vi "TxtToExcel v3.vi"() -> ()   [LabVIEW 2016]
panel:
  out "output array":string[][](array[string])
  out "error out":errorcluster
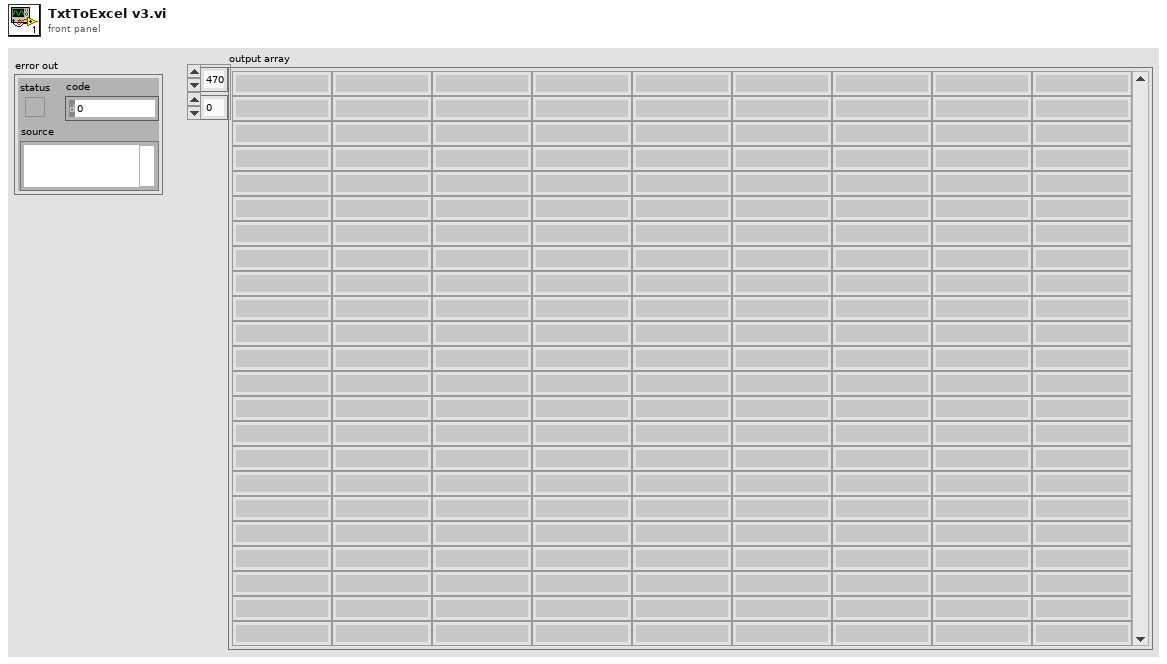
[diagram p1: front panel]
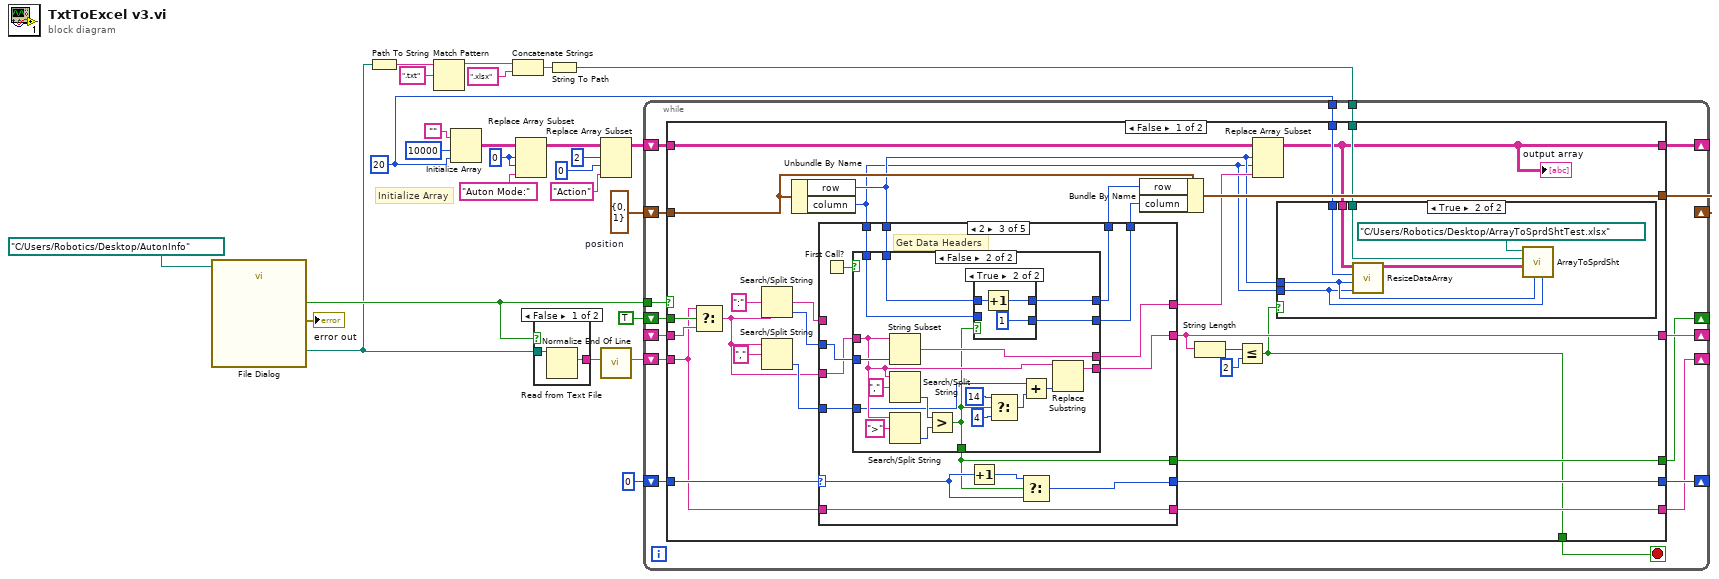
[diagram p0: block diagram]
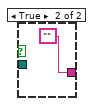
[diagram p2: hidden frame]
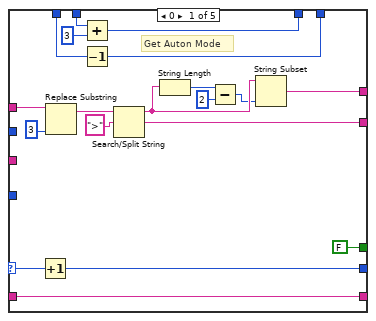
[diagram p4: hidden frame]
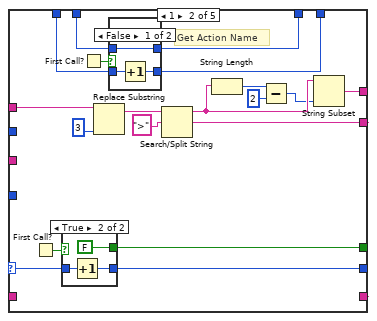
[diagram p5: hidden frame]
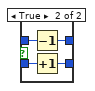
[diagram p6: hidden frame]
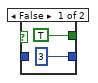
[diagram p7: hidden frame]
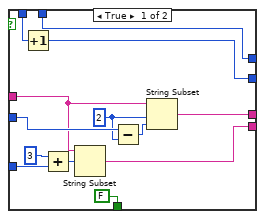
[diagram p8: hidden frame]
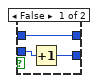
[diagram p9: hidden frame]
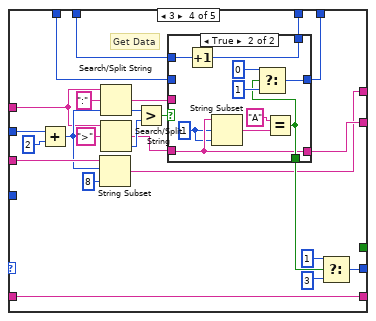
[diagram p10: hidden frame]
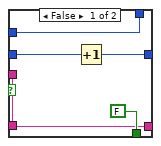
[diagram p11: hidden frame]
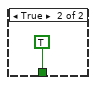
[diagram p13: hidden frame]
diagram:
  w15 = 0 ("index (row)")
  w17 = cluster{"row":i32, "column":i32} {"row"=0, "column"=1}  # position
  w1 = 20 ("Column Max")
  # "Initialize Array"
  n1 = call "File Dialog"("start path"=path "C:/Users/Robotics/Desktop/AutonInfo") -> ("selected path"=w8:path, "cancelled"=w24:bool, "error out"=→"error out":errorcluster)  [unwired: 11 in, 1 out]
  n2 = Path To String(path=w8) -> (string=w7:string)
  n3 = Match Pattern(string=w7, regular expression=".txt") -> (before substring=w3:string)  [unwired: 1 in, 3 out]
  n4 = Initialize Array("", 10000 ("Row Max"), w1) -> (w16:string[][])
  n5 = Concatenate Strings(w3, ".xlsx" ("string")) -> (w5:string)
  n6 = Replace Array Subset(array=w16, new element="Auton Mode:" ("new element/subarray"), index (row)=w15, index (col)=w15) -> (w13:string[][])
  n7 = case shown="False" w24 {
    tunnel: w8 -> [w28 _]
    tunnel: [w27 ""] -> w21
    frame False {
      n8 = Read from Text File(file (use dialog)=w28) -> (text=w27:string)  [unwired: 3 in, 3 out]
    }
    frame True {
    }
  }
  n9 = String To Path(string=w5) -> (path=w4:path)
  n10 = Replace Array Subset(array=w13, new element="Action" ("new element/subarray"), index (row)=2, index (col)=0 ("disabled index (col)")) -> (w9:string[][])
  n11 = call <vilib>:"Normalize End Of Line.vi"("string in"=w21) -> ("string out"=w20:string)  [unwired: 7 in]
  n12 = while {
    tunnel: w24 -> [w45]
    shift-right: [w42] -> _
    shift-left: _ -> [w44]
    shift-right: [w40] -> _
    shift-left: 0 -> [w41]
    shift-right: [w38] -> _
    shift-left: TRUE -> [w39]
    shift-right: [w37] -> _
    shift-left: w20 -> [w36]
    shift-right: [w32] -> _
    shift-left: w9 -> [w34]
    shift-right: [w33] -> _
    shift-left: w17 -> [w35]
    tunnel: w4 -> [w31]
    tunnel: w1 -> [w30]
    stop <- w43 stop-if-true
    n13 = case shown="False" w45 {
      tunnel: w44 -> [w66 _]
      tunnel: [w51 TRUE] -> w43
      tunnel: [w62 _] -> w42
      tunnel: w41 -> [w70 _]
      tunnel: [w69 _] -> w40
      tunnel: w39 -> [w64 _]
      tunnel: [w63 _] -> w38
      tunnel: [w59 _] -> w37
      tunnel: w36 -> [w58 _]
      tunnel: w35 -> [w56 _]
      tunnel: w34 -> [w55 _]
      tunnel: [w57 _] -> w33
      tunnel: [w46 _] -> w32
      tunnel: w31 -> [w50 _]
      tunnel: w30 -> [w47 _]
      frame False {
        n14 = Select(t=w58, s=w64, f=w66) -> (s? t:f=w65:string)
        n15 = Search/Split String(string=w65, search string/char (-)=":") -> (match + rest of string=w71:string, offset of match=w68:i32)  [unwired: 1 in, 1 out]
        n16 = Search/Split String(string=w65, search string/char (-)=",") -> (offset of match=w67:i32)  [unwired: 1 in, 2 out]
        n17 = Unbundle By Name(w56) -> ("row"=w49:i32, "column"=w48:i32)
        n18 = case shown="2" w70 {
          selector: w70 -> [w91 w106 w138 _ w225]
          tunnel: w71 -> [w81 w114 _ w183 _]
          tunnel: [w94 w113 w143 w188 _] -> w54
          tunnel: [w97 w110 w141 w189 _] -> w62
          tunnel: w49 -> [w93 w111 w140 w196 w223]
          tunnel: [w86 w109 w133 w195 w223] -> w53
          tunnel: w48 -> [w89 w112 w139 w199 w222]
          tunnel: [w85 w108 w132 w198 w222] -> w52
          tunnel: [w90 w107 w144 w192 w225] -> w69
          tunnel: w68 -> [_ _ w136 w206 _]
          tunnel: w67 -> [_ _ w142 _ _]
          tunnel: w65 -> [_ _ w131 w186 _]
          tunnel: [FALSE w104 w135 _ _] -> w63
          tunnel: [w87 w110 w134 w191 w224] -> w59
          tunnel: w58 -> [w87 _ w134 w191 w224]
          frame 0 {
            # "Get Auton Mode"
            n19 = Increment(x=w91) -> (x+1=w90:i32)
            n20 = Replace Substring(2:3 ("length (len. of substring)"), 5:w81) -> (1:w98:string)  [unwired: 2 in, 1 out]
            n21 = Add(x=w93, y=3) -> (x+y=w86:i32)
            n22 = Decrement(x=w89) -> (x-1=w85:i32)
            n23 = Search/Split String(string=w98, search string/char (-)=">") -> (substring before match=w95:string, match + rest of string=w97:string)  [unwired: 1 in, 1 out]
            n24 = String Length(string=w95) -> (length=w84:i32)
            n25 = Subtract(x=w84, y=2) -> (x-y=w83:i32)
            n26 = String Subset(string=w95, length (rest)=w83) -> (substring=w94:string)  [unwired: 1 in]
          }
          frame 1 {
            # "Get Action Name"
            n27 = First Call?() -> (First Call?: T/F=w105:bool)
            n28 = case shown="True" w105 {
              tunnel: [3 ("f") w130] -> w107
              tunnel: w106 -> [_ w129]
              tunnel: [TRUE FALSE] -> w104
              frame False {
              }
              frame True {
                n29 = Increment(x=w129) -> (x+1=w130:i32)
              }
            }
            n30 = First Call?() -> (First Call?: T/F=w103:bool)
            n31 = Replace Substring(2:3 ("length (len. of substring)"), 5:w114) -> (1:w117:string)  [unwired: 2 in, 1 out]
            n32 = case shown="False" w103 {
              tunnel: w112 -> [w121 w125]
              tunnel: w111 -> [w119 w124]
              tunnel: [w119 w123] -> w109
              tunnel: [w120 w122] -> w108
              frame False {
                n33 = Increment(x=w121) -> (x+1=w120:i32)
              }
              frame True {
                n34 = Decrement(x=w124) -> (x-1=w123:i32)
                n35 = Increment(x=w125) -> (x+1=w122:i32)
              }
            }
            n36 = Search/Split String(string=w117, search string/char (-)=">") -> (substring before match=w115:string, match + rest of string=w110:string)  [unwired: 1 in, 1 out]
            n37 = String Length(string=w115) -> (length=w100:i32)
            n38 = Subtract(x=w100, y=2) -> (x-y=w101:i32)
            n39 = String Subset(string=w115, length (rest)=w101) -> (substring=w113:string)  [unwired: 1 in]
          }
          frame 2 {
            # "Get Data Headers"
            n40 = First Call?() -> (First Call?: T/F=w137:bool)
            n41 = case shown="False" w137 {
              tunnel: w136 -> [w157 w172]
              tunnel: [w156 w176] -> w143
              tunnel: w142 -> [w154 w162]
              tunnel: [w153 w171] -> w141
              tunnel: [FALSE w161] -> w135
              tunnel: w140 -> [w147 w160]
              tunnel: [w147 w159] -> w133
              tunnel: w139 -> [w149 w174]
              tunnel: [w148 w173] -> w132
              tunnel: w131 -> [w146 w170]
              frame True {
                w155 = 2 ("length (len. of substring)")
                n42 = Increment(x=w149) -> (x+1=w148:i32)
                n43 = Add(x=3, y=w154) -> (x+y=w150:i32)
                n44 = String Subset(string=w146, offset (0)=w150) -> (substring=w153:string)  [unwired: 1 in]
                n45 = Subtract(x=w157, y=w155) -> (x-y=w158:i32)
                n46 = String Subset(string=w146, offset (0)=w155, length (rest)=w158) -> (substring=w156:string)
              }
              frame False {
                n47 = String Subset(string=w170, length (rest)=w172) -> (substring=w176:string)  [unwired: 1 in]
                n48 = Search/Split String(string=w170, search string/char (-)=",") -> (offset of match=w167:i32)  [unwired: 1 in, 2 out]
                n49 = Search/Split String(string=w170, search string/char (-)=">") -> (offset of match=w166:i32)  [unwired: 1 in, 2 out]
                n50 = Greater?(x=w167, y=w166) -> (0:w161:bool)
                n51 = case shown="True" w161 {
                  tunnel: w174 -> [w179 _]
                  tunnel: [w178 1] -> w173
                  tunnel: w160 -> [w177 w181]
                  tunnel: [w177 w180] -> w159
                  frame False {
                    n52 = Increment(x=w179) -> (x+1=w178:i32)
                  }
                  frame True {
                    n53 = Increment(x=w181) -> (x+1=w180:i32)
                  }
                }
                n54 = Select(t=14, s=w161, f=4) -> (s? t:f=w163:i32)
                n55 = Add(x=w162, y=w163) -> (x+y=w175:i32)
                n56 = Replace Substring(2:w175, 5:w170) -> (1:w171:string)  [unwired: 2 in, 1 out]
              }
            }
            n57 = Increment(x=w138) -> (x+1=w145:i32)
            n58 = Select(t=w145, s=w135, f=w138) -> (s? t:f=w144:i32)
          }
          frame 3 {
            # "Get Data"
            n59 = Add(x=w206, y=2) -> (x+y=w185:i32)
            n60 = String Subset(string=w186, offset (0)=w185, length (rest)=8 ("length (rest)")) -> (substring=w188:string)
            n61 = Search/Split String(string=w183, search string/char (-)=":", offset (0)=w185) -> (match + rest of string=w190:string, offset of match=w201:i32)  [unwired: 1 out]
            n62 = Search/Split String(string=w183, search string/char (-)=">") -> (match + rest of string=w184:string, offset of match=w200:i32)  [unwired: 1 in, 1 out]
            n63 = Greater?(x=w201, y=w200) -> (0:w197:bool)
            n64 = case shown="True" w197 {
              tunnel: w199 -> [w211 _]
              tunnel: [w210 w215] -> w198
              tunnel: w196 -> [w209 w219]
              tunnel: [w209 w218] -> w195
              tunnel: [FALSE w214] -> w194
              tunnel: w190 -> [w207 _]
              tunnel: w184 -> [_ w213]
              tunnel: [w207 w213] -> w189
              frame False {
                n65 = Increment(x=w211) -> (x+1=w210:i32)
              }
              frame True {
                w212 = 1 ("length (rest)")
                n66 = Increment(x=w219) -> (x+1=w218:i32)
                n67 = String Subset(string=w213, offset (0)=w212, length (rest)=w212) -> (substring=w221:string)
                n68 = Equal?(x="A", y=w221) -> (x = y?=w214:bool)
                n69 = Select(t=0 ("length (rest)"), s=w214, f=1 ("length (rest)")) -> (s? t:f=w215:i32)
              }
            }
            n70 = Select(t=1 ("length (rest)"), s=w194, f=3 ("length (rest)")) -> (s? t:f=w192:i32)
          }
          frame 4, Default {
          }
        }
        n71 = Bundle By Name(cluster=w56, "row"=w53, "column"=w52) -> (w57:cluster{"row":i32, "column":i32})
        n72 = String Length(string=w62) -> (length=w61:i32)
        n73 = Less Or Equal?(x=w61, y=2) -> (x <= y?=w51:bool)
        n74 = Replace Array Subset(array=w55, new element=w54, index (row)=w49, index (col)=w48) -> (w46:string[][])
        "output array" <- w46
        n75 = case shown="True" w51 {
          tunnel: w46 -> [_ w78]
          tunnel: w50 -> [_ w79]
          tunnel: w49 -> [_ w75]
          tunnel: w48 -> [_ w74]
          tunnel: w47 -> [_ w77]
          frame False {
          }
          frame True {
            n76 = call "ResizeDataArray.vi"("Column"=w74, "Row"=w75, "Column Max"=w77, "Input Array"=w78) -> ("Output Array"=w76:string[][])  [unwired: 3 in]
            n77 = call "ArrayToSprdSht.vi"("Column End"=w74, "Row End"=w75, "TextArray"=w76, "report file path"=w79, "template (empty)"=path "C:/Users/Robotics/Desktop/ArrayToSprdShtTest.xlsx" ("file path (dialog if empty)")) -> ()  [unwired: 7 in]
          }
        }
      }
      frame True {
      }
    }
  }
